vi "P4CMDSub ClientsString to ClientList.vi"(1 "users string":string) -> (0 "users list":string[][](array[string]))   [LabVIEW 2020, in "NI_SCC_P4CMD.lvlib"]
uses:
  <vilib>/SourceControl/Providers/P4CMD/NI_SCC_P4CMD.lvlib
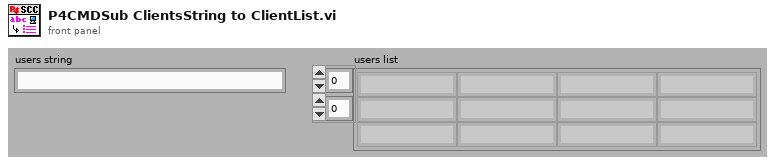
[diagram p1: front panel]
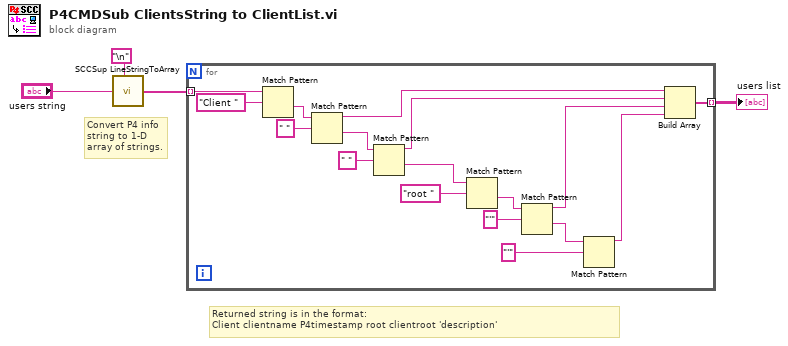
[diagram p0: block diagram]
diagram:
  # "Convert P4 info string to 1-D array of strings."
  # "Returned string is in the format:\nClient clientname P4timestamp root clientroot 'description'"
  n1 = call <vilib>:"SCCSup LineStringToArray.vi"("delimiter (Tab)"="\n", "line string"="users string") -> ("line array"=w1:string[])  [unwired: 7 in]
  n2 = for {
    tunnel: w1 -> [w13] mode=indexing
    tunnel: [w21] -> w4 mode=indexing
    n3 = Match Pattern(string=w13, regular expression="Client ") -> (after substring=w18:string)  [unwired: 1 in, 3 out]
    n4 = Match Pattern(string=w18, regular expression=" ") -> (before substring=w9:string, after substring=w11:string)  [unwired: 1 in, 2 out]
    n5 = Match Pattern(string=w11, regular expression=" ") -> (before substring=w8:string, after substring=w10:string)  [unwired: 1 in, 2 out]
    n6 = Match Pattern(string=w10, regular expression="root ") -> (after substring=w17:string)  [unwired: 1 in, 3 out]
    n7 = Match Pattern(string=w17, regular expression="'") -> (before substring=w15:string, after substring=w14:string)  [unwired: 1 in, 2 out]
    n8 = Match Pattern(string=w14, regular expression="'") -> (before substring=w5:string)  [unwired: 1 in, 3 out]
    n9 = Build Array(w9, w8, w15, w5) -> (w21:string[])
  }
  "users list" <- w4
